vi "AudioTest.Select Device and Play_Record Audio.vi"(7 "Amplitude":dbl=0.9, 8 "error in":errorcluster, 9 "Rec Setup":T1={"Device"="", "Left En"=TRUE, "Right En"=TRUE, "PrePlaySec"=0.1, "PostPlaySec"=0.1}, 10 "Play Setup":T2={"Device"="", "Left En"=TRUE, "Right En"=TRUE, "Volume(%)"=50.0, "Amplitude"=1.0}, 11 "Play Wvfrm":waveform(dbl)[](graph)) -> (0 "error out":errorcluster, 3 "Rec Wvfrm":waveform(dbl)[](graph))   [LabVIEW 2018]
uses:
  Audio.Play Signal Setup.ctl
  Audio.Record Signal Setup.ctl
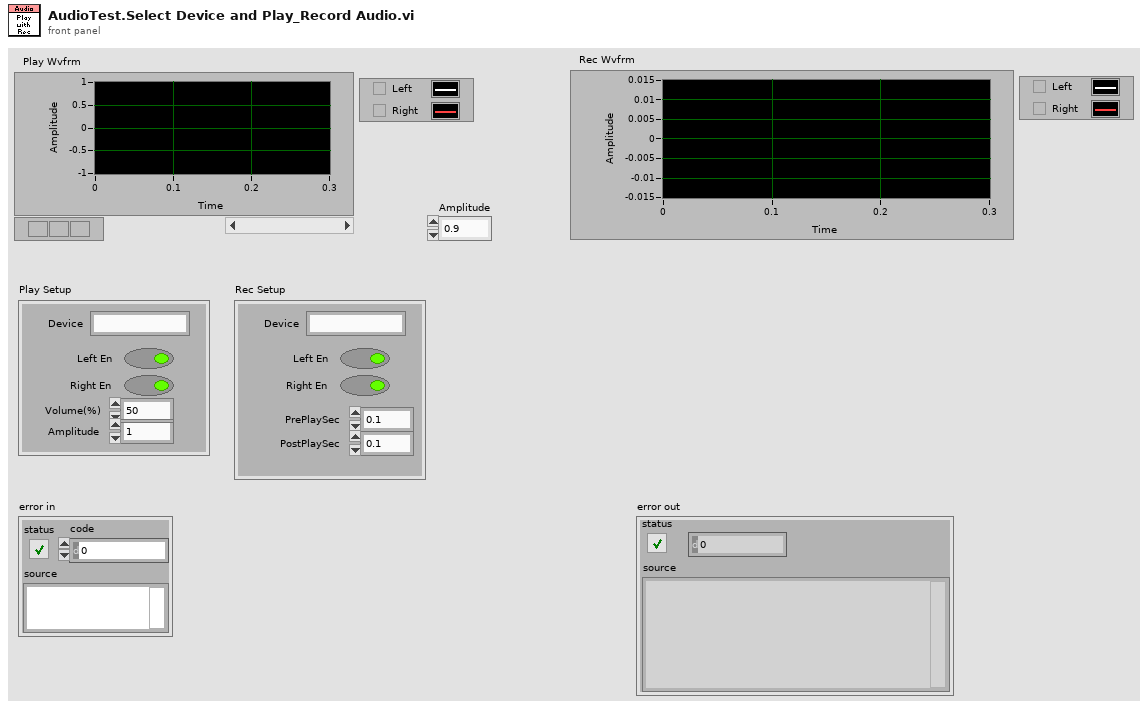
[diagram p1: front panel]
types:
  T1 = typedef "Audio.Record Signal Setup.ctl" = cluster{"Device":string, "Left En":bool, "Right En":bool, "PrePlaySec":dbl, "PostPlaySec":dbl}
  T2 = typedef "Audio.Play Signal Setup.ctl" = cluster{"Device":string, "Left En":bool, "Right En":bool, "Volume(%)":dbl, "Amplitude":dbl}
  T3 = cluster{"In ID":i32, "Out ID":i32, "Play Wvfrm":waveform(dbl)[], "Rec Wvfrm":waveform(dbl)[]}
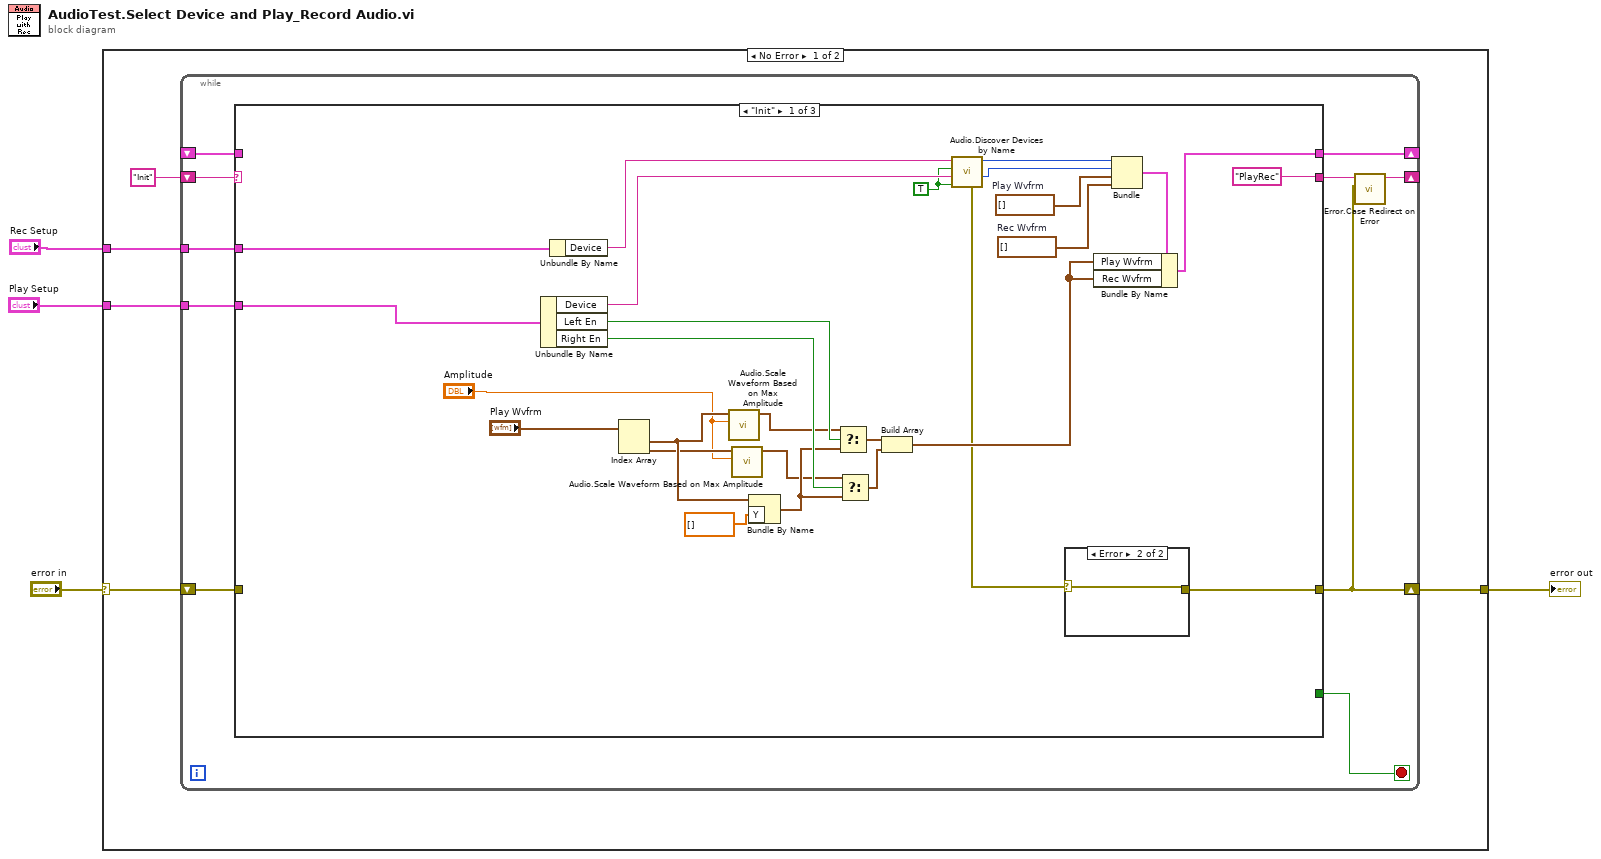
[diagram p0: block diagram]
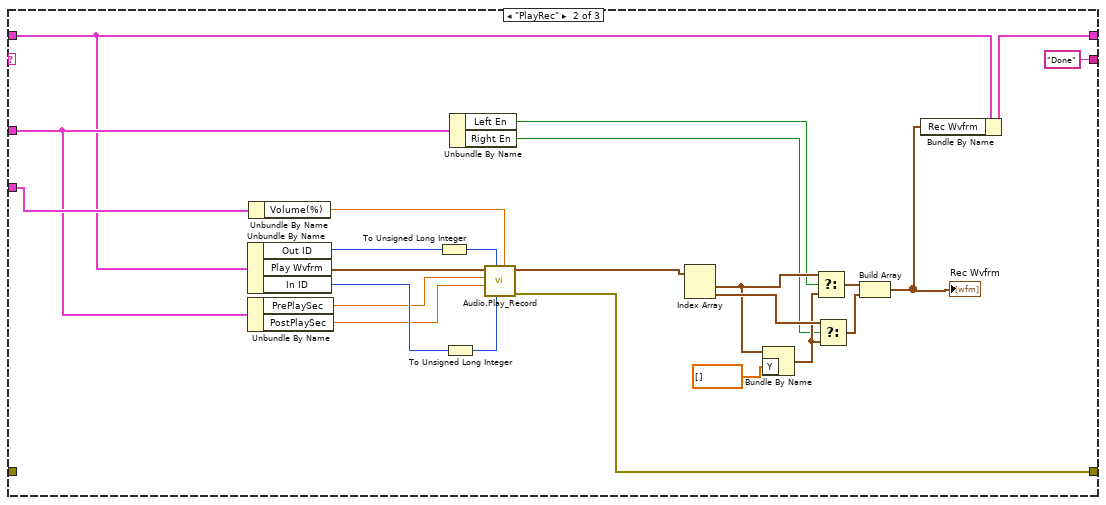
[diagram p3: hidden frame]
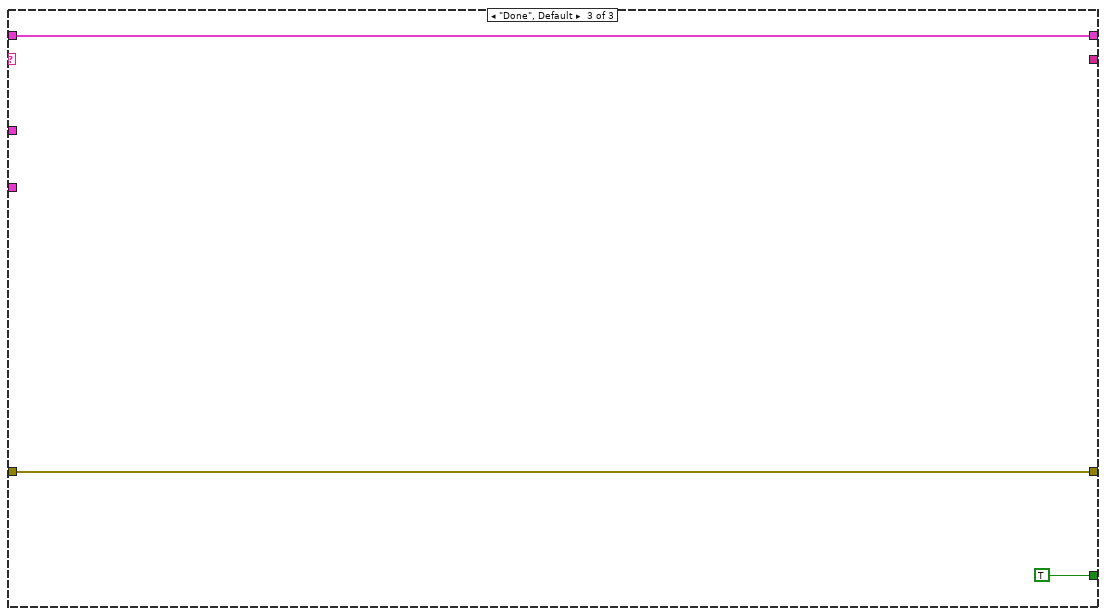
[diagram p4: hidden frame]
diagram:
  n1 = case shown="No Error" "error in" {
    selector: "error in" -> [w8 w76]
    tunnel: [w7 w76] -> w3
    tunnel: "Rec Setup" -> [w6 _]
    tunnel: "Play Setup" -> [w5 _]
    frame No Error {
      n2 = while {
        shift-right: [w11] -> _
        shift-left: _ -> [w18]
        tunnel: w6 -> [w14]
        tunnel: w5 -> [w13]
        shift-right: [w12] -> _
        shift-left: "Init" -> [w19]
        shift-right: [w16] -> w7
        shift-left: w8 -> [w17]
        stop <- w15 stop-if-true
        n3 = case shown="\"Init\"" w19 {
          tunnel: w18 -> [_ w50 w75]
          tunnel: [w32 w51 w75] -> w11
          tunnel: w17 -> [_ _ w73]
          tunnel: [w21 w63 w73] -> w16
          tunnel: [_ _ TRUE] -> w15
          tunnel: w14 -> [w46 w61 _]
          tunnel: w13 -> [w45 w65 _]
          tunnel: ["PlayRec" "Done" _] -> w10
          frame "Init" {
            w29 = waveform(dbl)[] []  # Rec Wvfrm
            w39 = waveform(dbl)[] []  # Play Wvfrm
            w42 = TRUE ("Error if In Dev Not Found")
            n4 = Unbundle By Name(w45) -> ("Device"=w43:string, "Left En"=w35:bool, "Right En"=w36:bool)
            n5 = Unbundle By Name(w46) -> ("Device"=w44:string)
            n6 = Index Array(array="Play Wvfrm") -> (element #1=w27:waveform(dbl), element #2=w25:waveform(dbl))  [unwired: 2 in]
            n7 = call "Audio.Scale Waveform Based on Max Amplitude.vi"("Max Amplitude"="Amplitude", "Wvfrm In"=w27) -> ("Wvfrm Out"=w26:waveform(dbl))  [unwired: 9 in]
            n8 = call "Audio.Scale Waveform Based on Max Amplitude.vi"("Max Amplitude"="Amplitude", "Wvfrm In"=w25) -> ("Wvfrm Out"=w24:waveform(dbl))  [unwired: 9 in]
            n9 = Bundle By Name(cluster=w27, "Y"=dbl[] []) -> (w30:waveform(dbl))
            n10 = Select(t=w26, s=w35, f=w30) -> (s? t:f=w37:waveform(dbl))
            n11 = Select(t=w24, s=w36, f=w30) -> (s? t:f=w34:waveform(dbl))
            n12 = Build Array(w37, w34) -> (w23:waveform(dbl)[])
            n13 = call "Audio.Discover Devices by Name.vi"("Error if Out Dev Not Found"=w42, "Output Device"=w43, "Error if In Dev Not Found"=w42, "Input Device"=w44) -> ("Out ID"=w40:i32, "In ID"=w41:i32, "error out"=w22:errorcluster)  [unwired: 3 in, 2 out]
            n14 = case shown="Error" w22 {
              selector: w22 -> [w47 w48]
              tunnel: [w47 w48] -> w21
              frame No Error {
              }
              frame Error {
              }
            }
            n15 = Bundle("In ID"=w41, "Out ID"=w40, "Play Wvfrm"=w39, "Rec Wvfrm"=w29) -> (w33:T3)  [unwired: 1 in]
            n16 = Bundle By Name(cluster=w33, "Play Wvfrm"=w23, "Rec Wvfrm"=w23) -> (w32:T3)
          }
          frame "PlayRec" {
            n17 = Unbundle By Name(w50) -> ("Out ID"=w71:i32, "Play Wvfrm"=w72:waveform(dbl)[], "In ID"=w69:i32)
            n18 = Unbundle By Name(w61) -> ("PrePlaySec"=w67:dbl, "PostPlaySec"=w66:dbl)
            n19 = Unbundle By Name(w65) -> ("Volume(%)"=w64:dbl)
            n20 = To Unsigned Long Integer(number=w71) -> (unsigned 32bit integer=w70:u32)
            n21 = To Unsigned Long Integer(number=w69) -> (unsigned 32bit integer=w68:u32)
            n22 = Unbundle By Name(w61) -> ("Left En"=w52:bool, "Right En"=w53:bool)
            n23 = call "Audio.Play_Record.vi"("volume"=w64, "Record Device ID"=w68, "Play Device ID"=w70, "RcdPostTime"=w66, "RcdPreTime"=w67, "Play Wvfrm"=w72) -> ("Error Out"=w63:errorcluster, "Rcd Wvfrm"=w54:waveform(dbl)[])  [unwired: 3 in, 1 out]
            n24 = Index Array(array=w54) -> (element #1=w57:waveform(dbl), element #2=w59:waveform(dbl))  [unwired: 2 in]
            n25 = Bundle By Name(cluster=w57, "Y"=dbl[] []) -> (w55:waveform(dbl))
            n26 = Select(t=w57, s=w52, f=w55) -> (s? t:f=w60:waveform(dbl))
            n27 = Select(t=w59, s=w53, f=w55) -> (s? t:f=w58:waveform(dbl))
            n28 = Build Array(w60, w58) -> (w49:waveform(dbl)[])
            "Rec Wvfrm" <- w49
            n29 = Bundle By Name(cluster=w50, "Rec Wvfrm"=w49) -> (w51:T3)
          }
          frame "Done", Default {
          }
        }
        n30 = call "Error.Case Redirect on Error.vi"("error in"=w16, "Next Case"=w10) -> ("Next Case Out"=w12:string)  [unwired: 9 in]
      }
    }
    frame Error {
    }
  }
  "error out" <- w3
